vi "Format S-parameters Graph.vi"(5 "S-parameter reference":refnum<vi>, 7 "Format":u16(ring) items=["Ampl (dB)", "Ampl (mag)", "Phase (deg)", "Phase (rad)", "Re", "Im"], 8 "error in (no error)":errorcluster, 9 "S-parameter Index":u16, 10 "Frequencies":dbl[](array[numeric]), 11 "S-parameters":cdb[][](array[numeric])) -> (0 "error out":errorcluster, 3 "S-parameter Graph":T1)   [LabVIEW 2023, in "NI_HFNetworkAnalysis.lvlib"]
doc: "Formats an S-parameter for plotting on an XY graph."
uses:
  NI_HFNetworkAnalysis.lvlib
  Controls/Quantity.ctl
  Controls/Unit.ctl
  Support VIs/Convert Unit (CDB Array).vi
  Support VIs/Convert Unit (DBL Array).vi
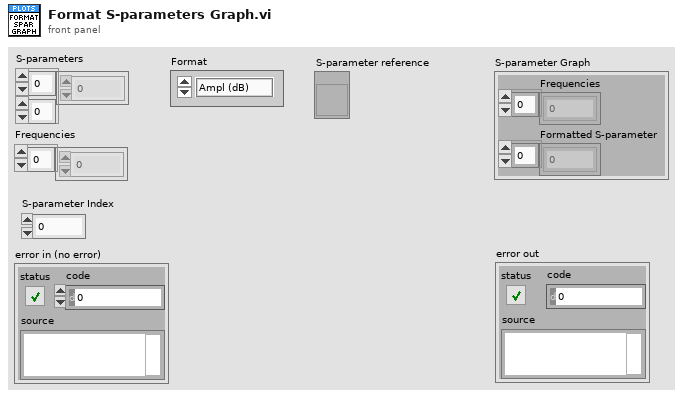
[diagram p1: front panel]
types:
  T1 = cluster{"Frequencies":dbl[], "Formatted S-parameter":dbl[]}
  T2 = typedef "NI_HFNetworkAnalysis.lvlib/Unit.ctl" = enum16{"No", "s", "Hz", "V", "A", "Ohm", "W", "dB", "dBV", "dBA", "dBm", "percent", "rad", "deg"}
  T3 = typedef "NI_HFNetworkAnalysis.lvlib/Quantity.ctl" = enum16{"Undefined", "V", "I", "A", "B", "P", "Z", "PowerRatio", "Gamma", "Index"}
  T4 = cluster{"FreqList":dbl[], "Converted Data":dbl[]}
  T5 = cluster{"Frequencies":dbl[], "Converted Data":dbl[]}
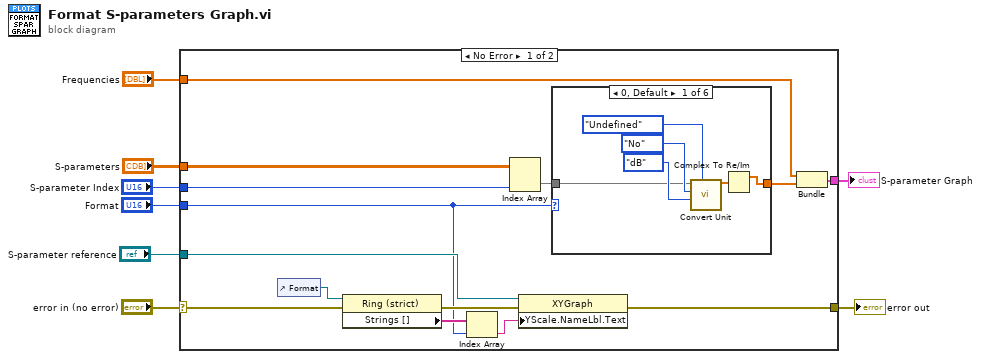
[diagram p0: block diagram]
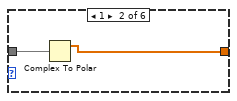
[diagram p2: hidden frame]
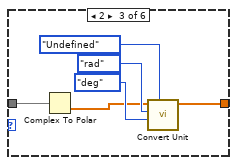
[diagram p3: hidden frame]
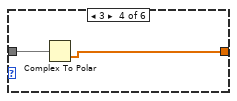
[diagram p4: hidden frame]
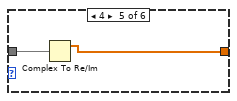
[diagram p5: hidden frame]
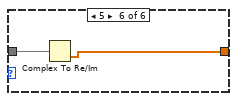
[diagram p6: hidden frame]
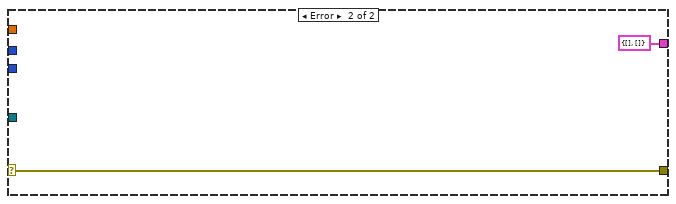
[diagram p7: hidden frame]
diagram:
  n1 = case shown="No Error" "error in (no error)" {
    selector: "error in (no error)" -> [w10 w44]
    tunnel: [w22 w44] -> w8
    tunnel: "S-parameters" -> [w20 _]
    tunnel: [w17 T4 {"FreqList"=[], "Converted Data"=[]}] -> w6
    tunnel: "S-parameter reference" -> [w16 _]
    tunnel: "Frequencies" -> [w15 _]
    tunnel: "S-parameter Index" -> [w12 _]
    tunnel: "Format" -> [w11 _]
    frame No Error {
      n2 = control-ref of="Format"() -> (w9:refnum<vi>)
      n3 = property on="Property Node" class="Ring (strict)"(reference=w9, error in=w10) -> (error out=w21:errorcluster, "Strings []"=w14:string[])  [unwired: 1 out]
      n4 = Index Array(array=w14, index=w11) -> (element=w13:string)
      n5 = Index Array(array=w20, index (col)=w12) -> (element=w18:cdb[])  [unwired: 1 in]
      n6 = property on="Property Node" class="XYGraph"(reference=w16, error in=w21, "YScale.NameLbl.Text"=w13) -> (error out=w22:errorcluster)  [unwired: 1 out]
      n7 = case shown="0, Default" w11 {
        tunnel: w18 -> [w25 w30 w32 w38 w40 w42]
        tunnel: [w23 w29 w33 w37 w39 w41] -> w19
        frame 0, Default {
          n8 = call-poly "Convert Unit.vi"("Quantity"=Quantity."Undefined", "Target Unit"=Unit."dB", "Base Unit"=Unit."No", "Data"=w25) -> ("Converted Data"=w24:cdb[])  [unwired: 3 in, 1 out]
          n9 = Complex To Re/Im(x + iy=w24) -> (x=w23:dbl[])  [unwired: 1 out]
        }
        frame 1 {
          n10 = Complex To Polar(r * e^(i*theta)=w30) -> (r=w29:dbl[])  [unwired: 1 out]
        }
        frame 2 {
          n11 = Complex To Polar(r * e^(i*theta)=w32) -> (theta=w31:dbl[])  [unwired: 1 out]
          n12 = call-poly "Convert Unit.vi"("Quantity"=Quantity."Undefined", "Target Unit"=Unit."deg", "Base Unit"=Unit."rad", "Data"=w31) -> ("Converted Data"=w33:dbl[])  [unwired: 3 in, 1 out]
        }
        frame 3 {
          n13 = Complex To Polar(r * e^(i*theta)=w38) -> (theta=w37:dbl[])  [unwired: 1 out]
        }
        frame 4 {
          n14 = Complex To Re/Im(x + iy=w40) -> (x=w39:dbl[])  [unwired: 1 out]
        }
        frame 5 {
          n15 = Complex To Re/Im(x + iy=w42) -> (y=w41:dbl[])  [unwired: 1 out]
        }
      }
      n16 = Bundle("Frequencies"=w15, "Converted Data"=w19) -> (w17:T5)  [unwired: 1 in]
    }
    frame Error {
    }
  }
  "error out" <- w8
  "S-parameter Graph" <- w6
